vi "MOV_XY_rotate.vi"(0 "System no.":i32=1 min=1 max=4 step=1, 2 "x state":dbl, 3 "y state":dbl, 5 "param":T1, 11 "error in":errorcluster) -> (4 "x target":dbl, 6 "y target":dbl, 8 "x num out":dbl, 10 "y num out":dbl, 15 "error out":errorcluster)   [LabVIEW 2013]
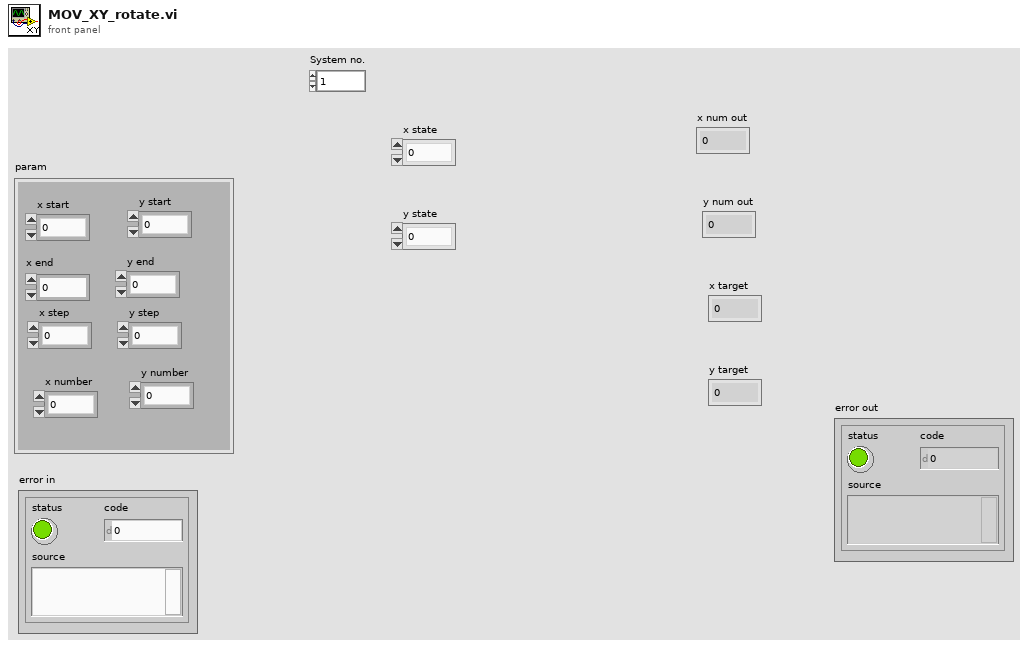
[diagram p1: front panel]
types:
  T1 = cluster{"x start":dbl, "y start":dbl, "y end":dbl, "x end":dbl, "x number":dbl, "y number":dbl, "y step":dbl, "x step":dbl}
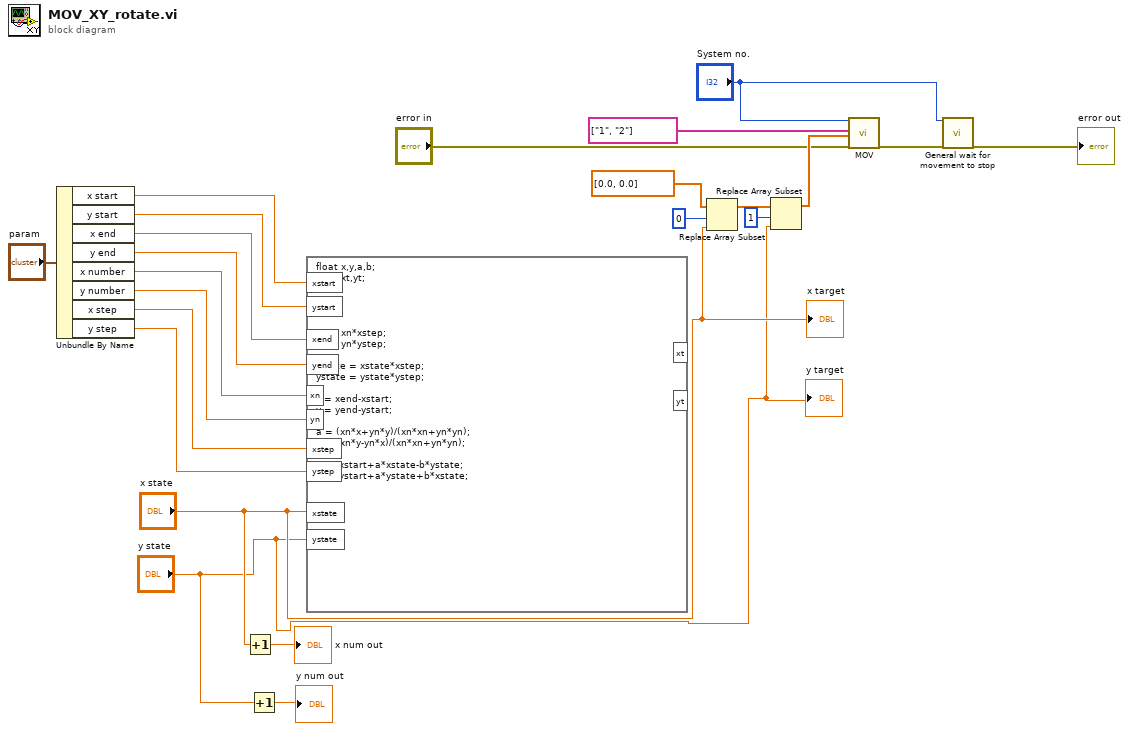
[diagram p0: block diagram]
diagram:
  n1 = Unbundle By Name("param") -> ("x start"=w10:dbl, "y start"=w9:dbl, "x end"=w8:dbl, "y end"=w7:dbl, "x number"=w6:dbl, "y number"=w5:dbl, "x step"=w4:dbl, "y step"=w3:dbl)
  n2 = Increment(x="x state") -> (x+1=→"x num out":dbl)
  n3 = Increment(x="y state") -> (x+1=→"y num out":dbl)
  n4 = formula code="float x,y,a,b;\nfloat xt,yt;\n\nxn--;\nyn--;\n\nxn = xn*xstep;\nyn = yn*ystep;\n\nxstate = xstate*xstep;\nystate = ystate*ystep;\n\nx = xend-xstart;\ny = yend-ystart;\n\na = (xn*x+yn*y)/(xn*xn+yn*yn);\nb = (xn*y-yn*x)/(xn*xn+yn*yn);\n\nxt = xstart+a*xstate-b*ystate;\nyt = ystart+a*ystate+b*xstate;"("xstart"=w10, "ystart"=w9, "xend"=w8, "yend"=w7, "xstate"="x state", "ystate"="y state", "xn"=w6, "yn"=w5, "xstep"=w4, "ystep"=w3) -> ()  [unwired: 2 out]
  n5 = Replace Array Subset(array=dbl[] [0.0, 0.0], new element="x state", index=0) -> (w20:dbl[])
  n6 = Replace Array Subset(array=w20, new element="y state", index=1) -> (w18:dbl[])
  n7 = call "MOV.vi"("System no."="System no.", "Axes to move"=string[] ["1", "2"], "Position values"=w18, "error in"="error in") -> ("error out"=w16:errorcluster)  [unwired: 15 in]
  n8 = call "General wait for movement to stop.vi"("System no."="System no.", "error in"=w16) -> ("error out"=→"error out":errorcluster)  [unwired: 16 in, 1 out]
  "x target" <- "x state"
  "y target" <- "y state"
